vi "Spinner Uninit.vi"(2 "Container State":T1, 3 "Display State":T2) -> ()   [LabVIEW 2012, in "Spinner.xctl"]
uses:
  Spinner.xctl
  Spinner State.ctl
  <vilib>/_xctls/Container State.ctl
  Command.ctl
  <vilib>/_xctls/XControlSupport.lvlib
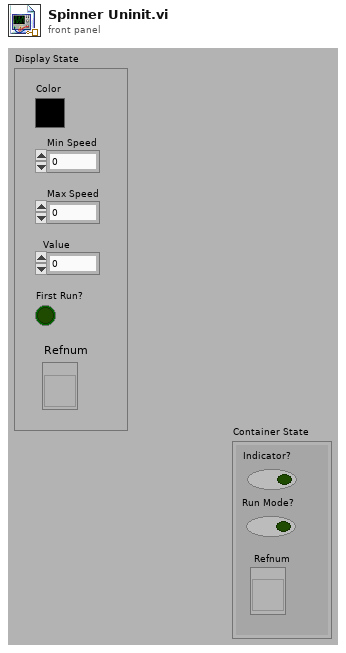
[diagram p1: front panel]
types:
  T1 = typedef "XControlSupport.lvlib/Container State.ctl" = cluster{"Indicator?":bool, "Run Mode?":bool, " Refnum":refnum<vi>}
  T2 = typedef "Spinner.xctl/Spinner State.ctl" = cluster{"Min Speed":dbl, "Color":u32, "Max Speed":dbl, "First Run?":bool, "Value":dbl, "Refnum":refnum<vi>}
  T3 = typedef "Spinner.xctl/Command.ctl" = enum16{"Add Control", "Remove Control", "Update Imgs", "Update Speed", "Refresh"}
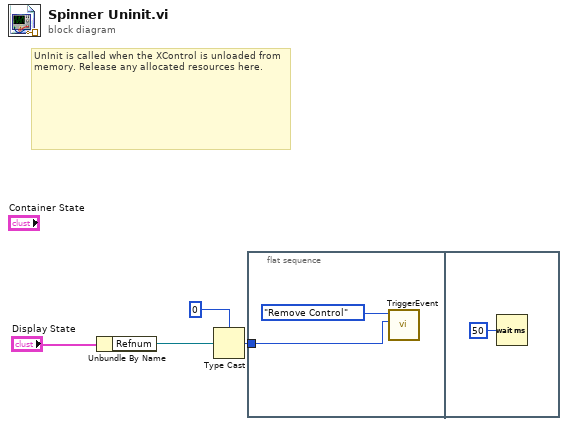
[diagram p0: block diagram]
diagram:
  # "UnInit is called when the XControl is unloaded from memory. Release any allocated resources here."
  n1 = Unbundle By Name("Display State") -> ("Refnum"=w1:refnum<vi>)
  n2 = Type Cast(type=u32 0, x=w1) -> (*(type *) &x=w3:u32)
  n3 = flat-sequence {
    tunnel: w3 -> [w6]
    frame #0 {
      n4 = call "TriggerEvent.vi"("Ctrl Ref"=w6, "Command"=Command."Remove Control") -> ()  [unwired: 9 in, 1 out]
    }
    frame #1 {
      n5 = Wait (ms)(milliseconds to wait=u32 50) -> ()  [unwired: 1 out]
    }
  }
